vi "DEMO.vi"(8 "errin":errorcluster, 10 "DATA IN":T1, 11 "table":string) -> (0 "error out":errorcluster)   [LabVIEW 2020]
uses:
  93f8419f-589b-4a81-b62e-70ffcd900bdb.vi
panel:
  out "chaîne concaténée":string
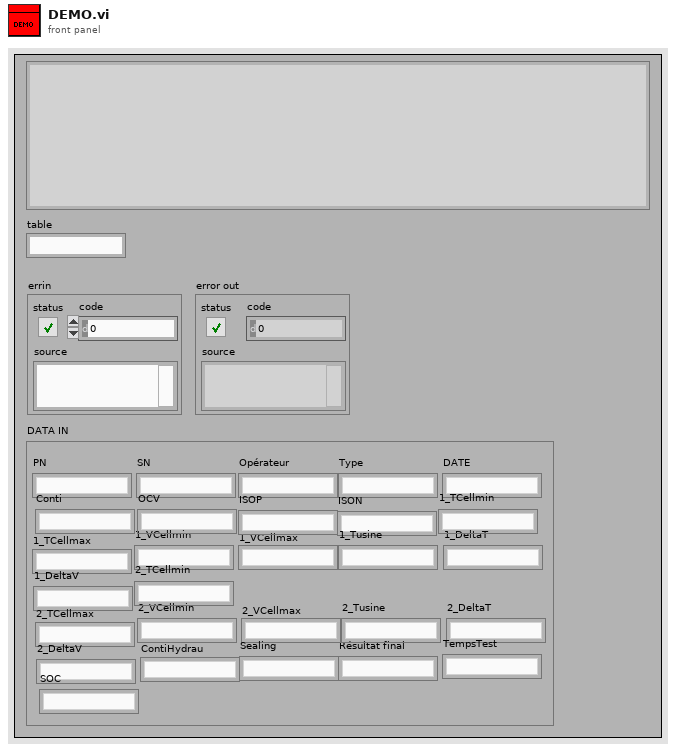
[diagram p1: front panel]
types:
  T1 = cluster{"PN":string, "SN":string, "Opérateur":string, "Type":string, "DATE":string, "Conti":string, "OCV":string, "ISOP":string, "ISON":string, "1_TCellmin":string, "1_TCellmax":string, "1_VCellmin":string, "1_VCellmax":string, "1_Tusine":string, "1_DeltaT":string, "1_DeltaV":string, "2_TCellmin":string, "2_TCellmax":string, "2_VCellmin":string, "2_VCellmax":string, "2_Tusine":string, "2_DeltaT":string, "2_DeltaV":string, "ContiHydrau":string, "Sealing":string, "Résultat final":string, "TempsTest":string, "SOC":string}
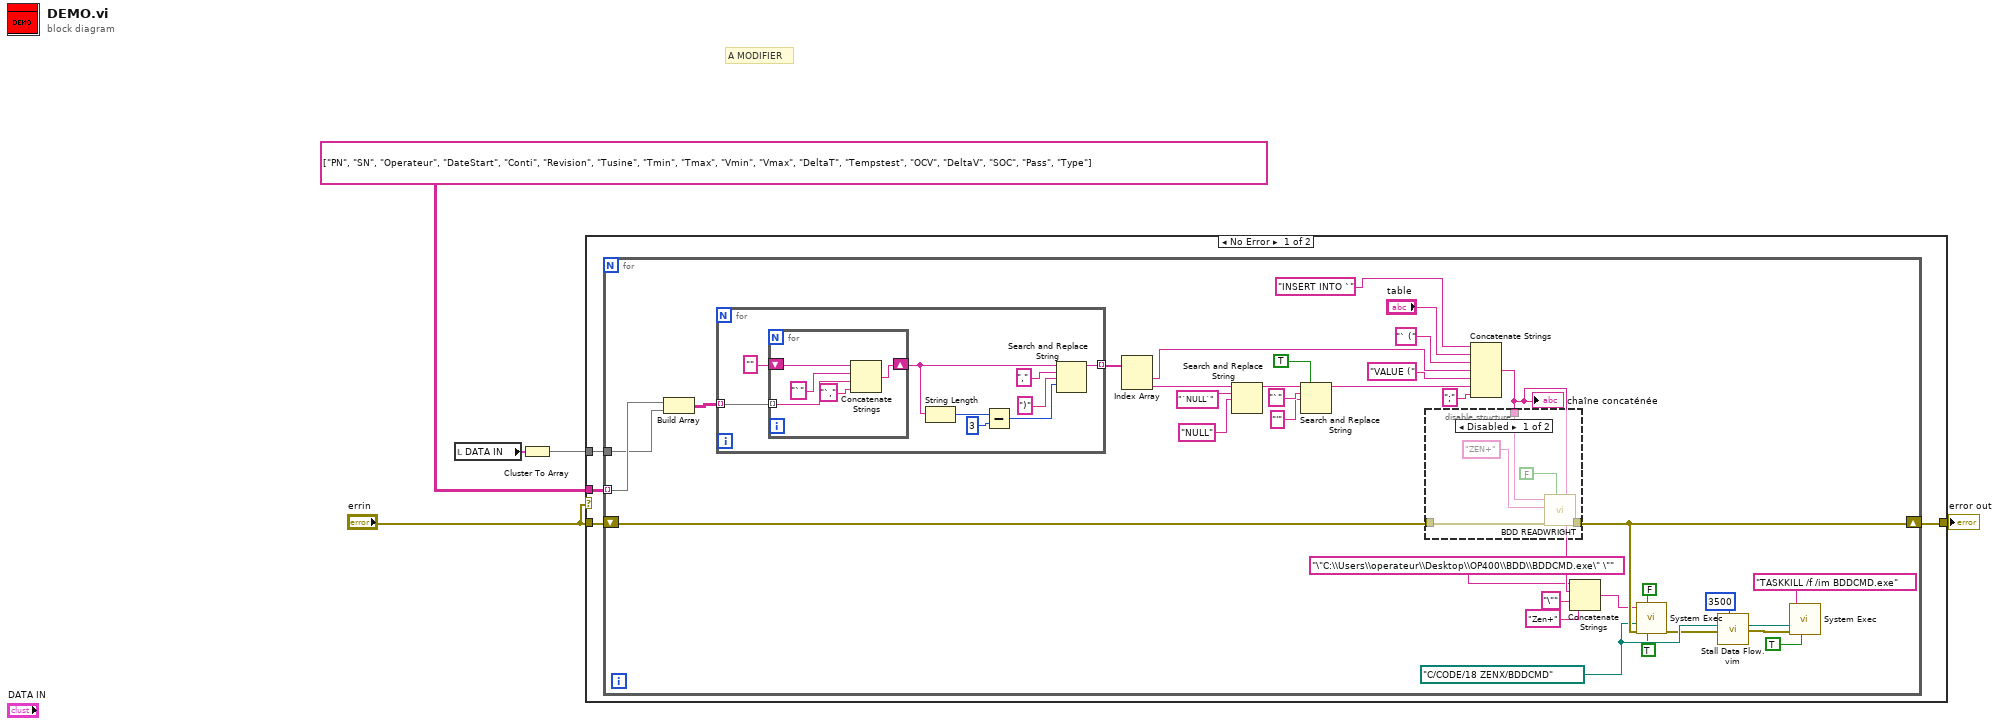
[diagram p0: block diagram]
diagram:
  # "A MODIFIER"
  n1 = local read "DATA IN"() -> (w1:T1)
  n2 = Cluster To Array(cluster=w1) -> (array=w2:string[])
  n3 = case shown="No Error" "errin" {
    tunnel: "errin" -> [w9 w62]
    tunnel: [w8 w62] -> w5
    tunnel: string[][] [["PN", "SN", "Operateur", "DateStart", "Conti", "Revision", "Tusine", "Tmin", "Tmax", "Vmin", "Vmax", "DeltaT", "Tempstest", "OCV", "DeltaV", "SOC", "Pass", "Type"]] -> [w7 _]
    tunnel: w2 -> [w6 _]
    frame No Error {
      n4 = for {
        shift-right: [w21] -> w8
        shift-left: w9 -> [w26]
        tunnel: w7 -> [w25] mode=indexing
        tunnel: w6 -> [w24]
        w19 = path "C:/CODE/18 ZENX/BDDCMD" ("working directory")
        n5 = Build Array(w25, w24) -> (w42:string[][])
        n6 = for {
          tunnel: [w48] -> w27 mode=indexing
          tunnel: w42 -> [w56] mode=indexing
          n7 = for {
            shift-right: [w59] -> w49
            shift-left: "" -> [w58]
            tunnel: w56 -> [w57] mode=indexing
            n8 = Concatenate Strings(w58, "`" ("string"), w57, "`," ("string")) -> (w59:string)
          }
          n9 = String Length(string=w49) -> (length=w54:i32)
          n10 = Subtract(x=w54, y=3) -> (x-y=w52:i32)
          n11 = Search and Replace String(input string=w49, search string=",", replace string=")" ("replace string (\"\")"), offset=w52) -> (result string=w48:string)  [unwired: 4 in, 3 out]
        }
        n12 = Index Array(array=w27) -> (element #1=w38:string, element #2=w39:string)  [unwired: 2 in]
        n13 = Search and Replace String(input string=w39, search string="`NULL`", replace string="NULL" ("replace string (\"\")")) -> (result string=w40:string)  [unwired: 5 in, 3 out]
        n14 = Search and Replace String(replace all?=TRUE ("replace all? (F)"), input string=w40, search string="`", replace string="'" ("replace string (\"\")")) -> (result string=w41:string)  [unwired: 4 in, 3 out]
        n15 = Concatenate Strings("INSERT INTO `" ("string"), "table", "` (" ("string"), w38, "VALUE (" ("string"), w41, ";" ("string")) -> (w23:string)
        "chaîne concaténée" <- w23
        n16 = disable-structure shown="Disabled" {
          disable-tunnel: w23 -> [w47 _]
          disable-tunnel: w26 -> [w46 _]
          disable-tunnel: [w45 _] -> w21
          frame Disabled {
            n17 = call <userlib>:"BDD READWRIGHT.vi"("Read?"=FALSE, "errin"=w46, "DSN name"="ZEN+", "Instruction"=w47) -> ("error out"=w45:errorcluster)  [unwired: 6 in, 1 out]
          }
          frame Enabled {
          }
        }
        n18 = Concatenate Strings("\"C:\\Users\\operateur\\Desktop\\OP400\\BDD\\BDDCMD.exe\" \"" ("string"), w23, "\"" ("string"), "Zen+" ("string")) -> (w16:string)
        n19 = call <vilib>:"System Exec.vi"("run minimized? (F)"=TRUE, "wait until completion? (T)"=FALSE, "error in (no error)"=w21, "working directory"=w19, "command line"=w16) -> ("error out"=w18:errorcluster)  [unwired: 3 in, 3 out]
        n20 = call "Stall Data Flow.vim"("value in"=w18, "milliseconds to wait"=u32 3500) -> ("value out"=w22:errorcluster)  [unwired: 1 out]
        n21 = call <vilib>:"System Exec.vi"("run minimized? (F)"=TRUE, "error in (no error)"=w22, "working directory"=w19, "command line"="TASKKILL /f /im BDDCMD.exe") -> ()  [unwired: 4 in, 4 out]
      }
    }
    frame Error {
    }
  }
  "error out" <- w5
